vi "BitfileDownloadedBroadcast_Parse.vi"(8 "error in (no error)":errorcluster, 11 "data":variant) -> (0 "error out":errorcluster, 3 "FPGA reference":refnum<k20>)   [LabVIEW 2017, in "FpgaBitfileManager.lvlib"]
uses:
  <vilib>/addons/InsightCM/Devices/Shared/Common/FpgaBitfileManager/FpgaBitfileManager.lvlib
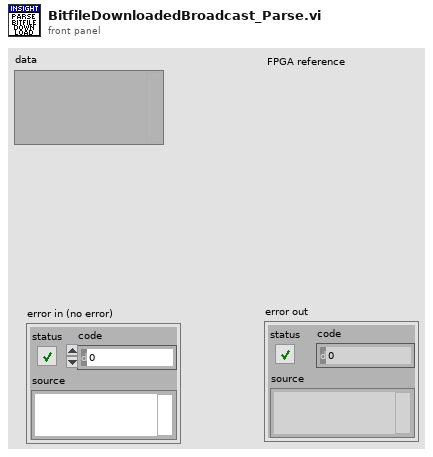
[diagram p1: front panel]
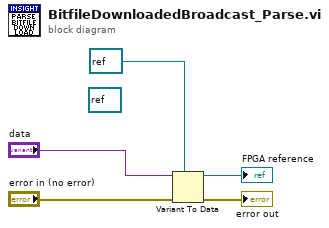
[diagram p0: block diagram]
diagram:
  (unwired) refnum<k20> refnum ("FPGA Interface")
  n1 = Variant To Data(error in="error in (no error)", type=refnum<k20> refnum ("Bitfile reference out"), Variant="data") -> (data=→"FPGA reference":refnum<k20>, error out=→"error out":errorcluster)
